vi "Destroy.vi"(0 "reference in":refnum<class "PartsTracking Controller.lvclass">, 5 "error in (no error)":errorcluster) -> (14 "reference out":refnum<class "PartsTracking Controller.lvclass">, 19 "error out":errorcluster)   [LabVIEW 2015, in "PartsTracking Controller.lvclass"]
doc: "Destructor."
uses:
  PartsTracking Controller.lvclass
  <vilib>/addons/_AddQ/G#Object/G#Object.lvclass
  APP/partsTracking_class/partsTracking.lvclass
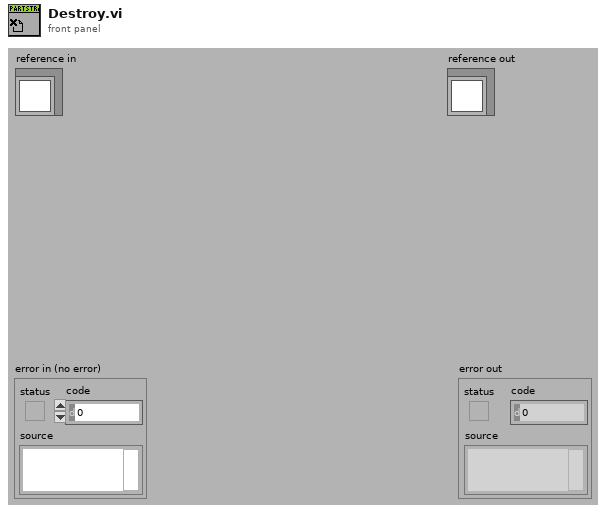
[diagram p1: front panel]
types:
  T1 = typedef "PartsTracking Controller.lvclass/ObjectAttributes.ctl" = cluster{"MyAttribute":dbl, "file_controller_ref":refnum<class "File Controller.lvclass">, "data":string[][], "partsTracking_ref":refnum<class "partsTracking.lvclass">, "project_panels_ref":refnum<class "Project Panels.lvclass">}
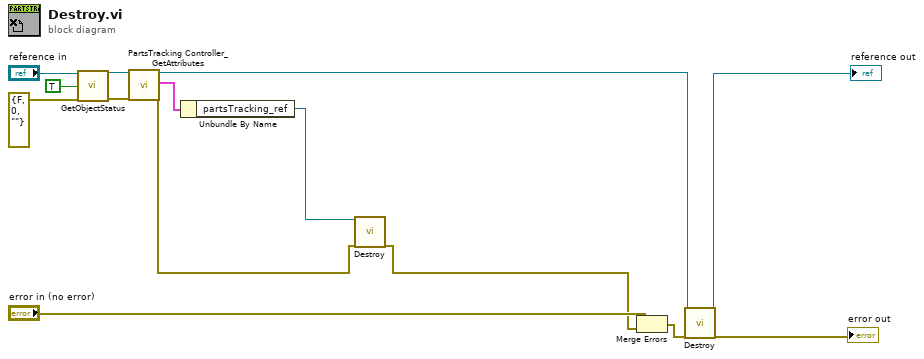
[diagram p0: block diagram]
diagram:
  n1 = call-dynamic "GetObjectStatus.vi"("reference in"="reference in", "simple info (F)"=TRUE ("simple info"), "error in (no error)"=errorcluster {"status"=FALSE, "code"=0, "source"=""}) -> ("reference out"=w8:refnum<class "PartsTracking Controller.lvclass">, "error out"=w9:errorcluster)  [unwired: 5 in, 10 out]
  n2 = call "PartsTracking Controller_GetAttributes.vi"("reference in"=w8, "error in (no error)"=w9) -> ("reference out"=w7:refnum<class "PartsTracking Controller.lvclass">, "attributes"=w6:T1, "error out"=w2:errorcluster)  [unwired: 14 in, 1 out]
  n3 = Unbundle By Name(w6) -> ("partsTracking_ref"=w3:refnum<class "partsTracking.lvclass">)
  n4 = call-dynamic "Destroy.vi"("reference in"=w3, "error in (no error)"=w2) -> ("error out"=w1:errorcluster)  [unwired: 16 in, 1 out]
  n5 = Merge Errors("error in (no error)", w1) -> (w13:errorcluster)
  n6 = call-parent "Destroy.vi"("reference in"=w7, "error in (no error)"=w13) -> ("reference out"=→"reference out":refnum<class "PartsTracking Controller.lvclass">, "error out"=→"error out":errorcluster)  [unwired: 16 in]
